vi "Save As Tiff.vi"(8 "error in (no error)":errorcluster, 11 "CCDCamera in":refnum<class "CCDCamera.lvclass">) -> (0 "error out":errorcluster, 3 "CCDCamera out":refnum<class "CCDCamera.lvclass">)   [LabVIEW 2018, in "CCDCamera.lvclass"]
doc: "Este VI salva a última imagem obtida pelo CCD no formato tiff."
uses:
  CCDCamera.lvclass
  CCDCamera.lvclass/CCDCamera.ctl
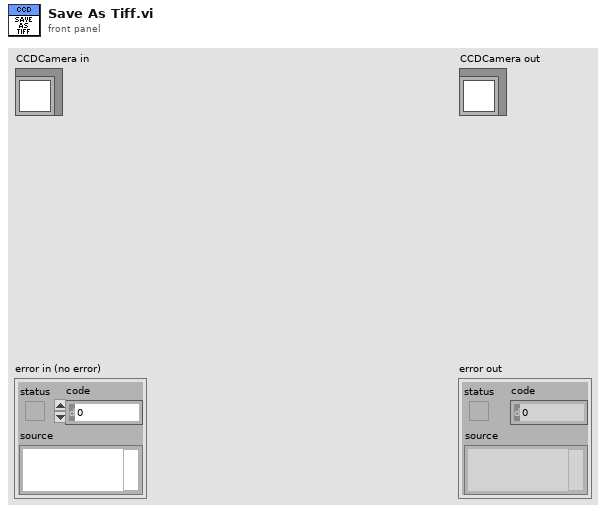
[diagram p1: front panel]
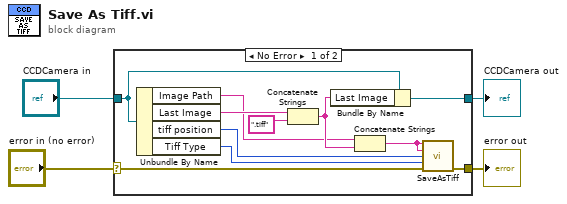
[diagram p0: block diagram]
diagram:
  n1 = case shown="No Error" "error in (no error)" {
    selector: "error in (no error)" -> [w15 w17]
    tunnel: [w14 w17] -> w3
    tunnel: [w10 w16] -> w1
    tunnel: "CCDCamera in" -> [w9 w16]
    frame No Error {
      n2 = Unbundle By Name(w9) -> ("Image Path"=w6:string, "Last Image"=w8:string, "tiff position"=w12:u16, "Tiff Type"=w13:u16)
      n3 = Concatenate Strings(w8, ".tiff") -> (w7:string)
      n4 = Bundle By Name(cluster=w9, "Last Image"=w7) -> (w10:refnum<class "CCDCamera.lvclass">)
      n5 = Concatenate Strings(w6, w7) -> (w5:string)
      n6 = call <userlib>:"SaveAsTiff.vi"("path"=w5, "palette"=w5, "position"=w12, "type"=w13, "error in (no error)"=w15) -> ("error out"=w14:errorcluster)  [unwired: 9 in, 1 out]
    }
    frame Error {
    }
  }
  "error out" <- w3
  "CCDCamera out" <- w1
